vi "Pop From Stack.vi"(8 "error in (no error)":errorcluster caption="错误输入（无错误）", 11 "Stack 输入":refnum<class "Stack.lvclass"> caption="DNL_LabVIEW Object in") -> (0 "error out":errorcluster caption="错误输出", 2 "Element":variant, 3 "Stack 输出":refnum<class "Stack.lvclass"> caption="DNL_LabVIEW Object out")   [LabVIEW 2011, in "Stack.lvclass"]
uses:
  Stack.lvclass
  Stack.lvclass/Stack.ctl
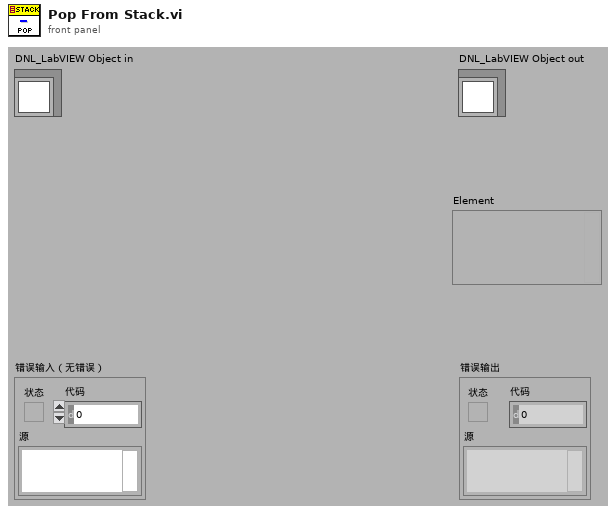
[diagram p1: front panel]
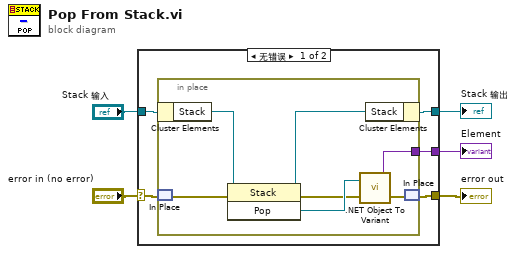
[diagram p0: block diagram]
diagram:
  n1 = case shown="无错误" "error in (no error)" {
    selector: "error in (no error)" -> [w7 w19]
    tunnel: [w6 w19] -> w4
    tunnel: [w9 w18] -> w2
    tunnel: "Stack 输入" -> [w10 w18]
    tunnel: [w8 _] -> w1
    frame No Error {
      n2 = in-place {
        in-place-border: [w13] -> w8
        n3 = in-place-cluster #1(w10) -> ("Stack"=w17:refnum<k24>)
        n4 = in-place-match #2(w7) -> (w12:errorcluster)
        n5 = invoke class="Stack" method="Pop"(reference=w17, error in=w12) -> (reference out=w16:refnum<k24>, error out=w14:errorcluster, "Pop"=w15:refnum<k24>)  [unwired: 1 in]
        n6 = call <vilib>:".NET Object To Variant.vi"("error in (no error)"=w14, ".NET object"=w15) -> ("error out"=w11:errorcluster, "variant"=w13:variant)
        n7 = in-place-cluster #1("Stack"=w16) -> (w9:refnum<class "Stack.lvclass">)
        n8 = in-place-match #2(w11) -> (w6:errorcluster)
      }
    }
    frame Error {
    }
  }
  "error out" <- w4
  "Stack 输出" <- w2
  "Element" <- w1
